vi "Calculate Side.vi"(8 "error in (no error)":errorcluster, 9 "Point 2":cluster{"X":dbl, "Y":dbl}, 10 "Point 1":cluster{"X":dbl, "Y":dbl}, 11 "Tool Rectangle in":refnum<class "Tool Rectangle.lvclass">) -> (0 "error out":errorcluster, 2 "Array":cluster{"X":dbl, "Y":dbl}[](array[cluster]), 3 "Tool Rectangle out":refnum<class "Tool Rectangle.lvclass">)   [LabVIEW 2019, in "Tool Rectangle.lvclass"]
uses:
  Tool Rectangle.lvclass
  Settings/Rectangle Settings/Rectangle Settings.lvclass/Rectangle Settings.ctl
  Settings/Rectangle Settings/Accessors/Read Fill Spacing.vi
  Settings/Rectangle Settings/Rectangle Settings.lvclass
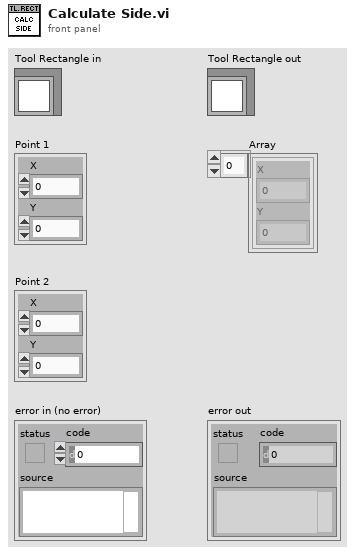
[diagram p1: front panel]
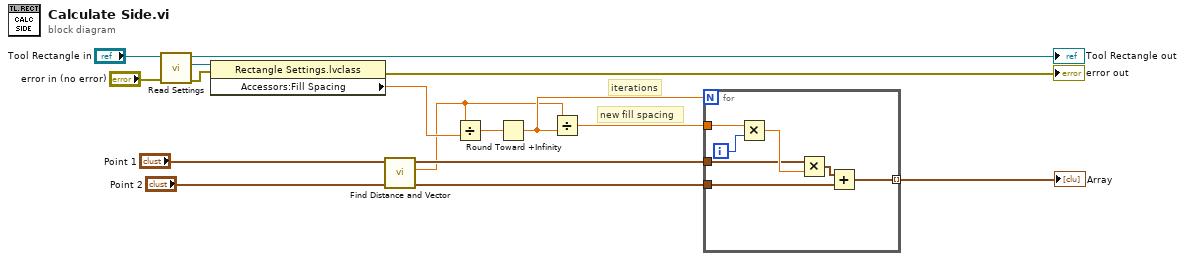
[diagram p0: block diagram]
diagram:
  # "new fill spacing"
  # "iterations"
  n1 = call-dynamic "Read Settings.vi"("error in (no error)"="error in (no error)", "Tool Rectangle in"="Tool Rectangle in") -> ("error out"=w5:errorcluster, "Rectangle Settings.lvclass"=w10:refnum<class "Rectangle Settings.lvclass">, "Tool Rectangle out"=→"Tool Rectangle out":refnum<class "Tool Rectangle.lvclass">)  [unwired: 7 in]
  n2 = property class="Rectangle Settings.lvclass"(reference=w10, error in=w5) -> (error out=→"error out":errorcluster, "Accessors:Fill Spacing"=w7:dbl)  [unwired: 1 out]
  n3 = call "Find Distance and Vector.vi"("Point 2"="Point 2", "Point 1"="Point 1") -> ("Distance"=w2:dbl, "Unit Vector"=w14:cluster{"X":dbl, "Y":dbl})  [unwired: 8 in]
  n4 = Divide(x=w2, y=w7) -> (x/y=w15:dbl)
  n5 = Round Toward +Infinity(x=w15) -> (ceil(x): smallest int >= x=w12:dbl)
  n6 = Divide(x=w2, y=w12) -> (x/y=w13:dbl)
  n7 = for {
    N: w12 -> [_]
    tunnel: w13 -> [w16]
    tunnel: "Point 2" -> [w19]
    tunnel: [w18] -> w1 mode=indexing
    tunnel: w14 -> [w17]
    i -> [w22]
    n8 = Multiply(x=w16, y=w22) -> (x*y=w21:dbl)
    n9 = Multiply(x=w17, y=w21) -> (x*y=w20:cluster{"X":dbl, "Y":dbl})
    n10 = Add(x=w20, y=w19) -> (x+y=w18:cluster{"X":dbl, "Y":dbl})
  }
  "Array" <- w1
